vi "niScope Direct DMA Fetch Binary.vi"(0 "instrument handle":refnum<k15>, 1 "timeout":dbl=5.0 format="%.2f", 5 "channels":string="0", 9 "numSamples":i32=-1, 11 "error in":errorcluster, 12 "bufferSize":u32, 13 "bufferAddress":u32) -> (4 "instrument handle out":refnum<k15>, 6 "wfm info":T1 {"reserved2" format="%.2f"; "reserved1" format="%.2f"; "offset" format="%^.3e"; "gain" format="%^.3e"; "xIncrement" format="%^.3e"; "relativeInitialX" format="%^.3e"; "absoluteInitialX" format="%^.3e"}, 10 "offsetToFirstSample":i32, 15 "error out":errorcluster)   [LabVIEW 2013]
uses:
  niScope_32.dll
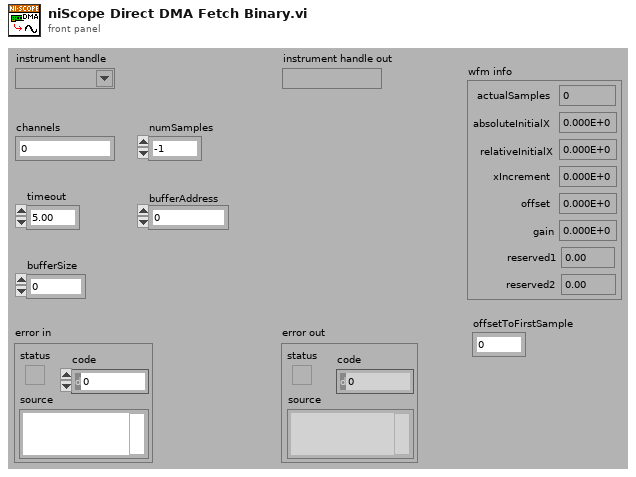
[diagram p1: front panel]
types:
  T1 = cluster{"actualSamples":i32, "absoluteInitialX":dbl, "relativeInitialX":dbl, "xIncrement":dbl, "offset":dbl, "gain":dbl, "reserved1":dbl, "reserved2":dbl}
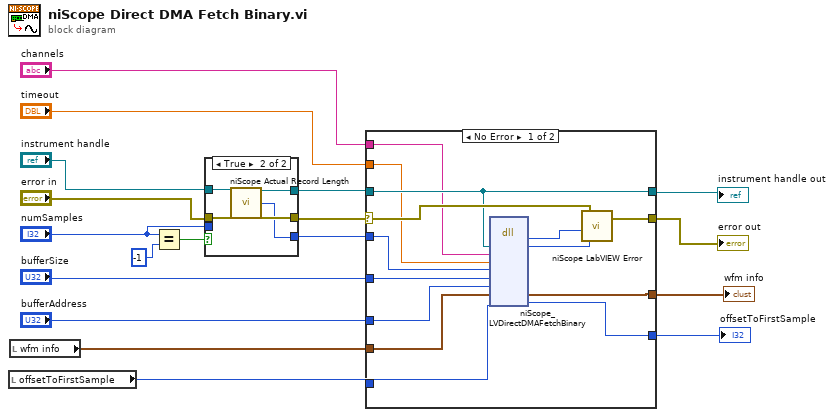
[diagram p0: block diagram]
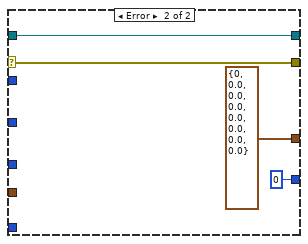
[diagram p3: hidden frame]
diagram:
  n1 = local read "offsetToFirstSample"() -> (w4:i32)
  n2 = local read "wfm info"() -> (w1:T1)
  n3 = Equal?(x="numSamples", y=-1) -> (x = y?=w15:bool)
  n4 = case shown="True" w15 {
    tunnel: [w20 w26] -> w12
    tunnel: [w21 w25] -> w13
    tunnel: "numSamples" -> [w19 _]
    tunnel: [w19 w22] -> w11
    tunnel: "instrument handle" -> [w21 w24]
    tunnel: "error in" -> [w20 w23]
    frame False {
    }
    frame True {
      n5 = call <instrlib>:"niScope Actual Record Length.vi"("instrument handle"=w24, "error in"=w23) -> ("instrument handle out"=w25:refnum<k15>, "actual record length"=w22:i32, "error out"=w26:errorcluster)  [unwired: 11 in]
    }
  }
  n6 = case shown="No Error" w12 {
    selector: w12 -> [w37 w43]
    tunnel: [w38 w43] -> w18
    tunnel: w13 -> [w36 w44]
    tunnel: [w36 w44] -> w17
    tunnel: w11 -> [w33 _]
    tunnel: [w27 T1 {"actualSamples"=0, "absoluteInitialX"=0.0, "relativeInitialX"=0.0, "xIncrement"=0.0, "offset"=0.0, "gain"=0.0, "reserved1"=0.0, "reserved2"=0.0} ("wfm info")] -> w2
    tunnel: "timeout" -> [w35 _]
    tunnel: "channels" -> [w34 _]
    tunnel: "bufferSize" -> [w32 _]
    tunnel: [w31 0 ("offsetToFirstSample")] -> w5
    tunnel: w4 -> [w30 _]
    tunnel: "bufferAddress" -> [w29 _]
    tunnel: w1 -> [w28 _]
    frame No Error {
      n7 = dll-call lib="niScope_*.*" fn="niScope_LVDirectDMAFetchBinary"("instrument handle"=w36, "channel"=w34, "timeout"=w35, "numSamples"=w33, "bufferSize"=w32, "bufferAddress"=w29, "wfm_info"=w28, "offsetToFirstSample"=w30) -> ("status"=w40:i32, "instrument handle"=w39:u32, "wfm_info"=w27:T1, "offsetToFirstSample"=w31:i32)  [unwired: 8 in, 2 out]
      n8 = call <instrlib>:"niScope LabVIEW Error.vi"("instrument handle"=w39, "niScope error code (0)"=w40, "error in (no error)"=w37) -> ("error out"=w38:errorcluster)  [unwired: 2 in]
    }
    frame Error {
    }
  }
  "instrument handle out" <- w17
  "error out" <- w18
  "offsetToFirstSample" <- w5
  "wfm info" <- w2
